vi "create.volume.filename.vi"(11 "volume":T1={"id"=0, "name"="", "sortable_name"="", "aliases"=[], "description"="", "site_detail_url"="", "count_of_issues"=0, "start_year"=0, "publisher_id"=0, "issue_ids"=[], "date_last_updated"=timestamp(0 s since 1904-01-01), "volume"=0, "cv_id"="", "volume type"=enum."One Shot"}) -> (3 "json filename":string)   [LabVIEW 2024]
uses:
  definitions/local_volume.ctl
  definitions/volume.type--enum.ctl
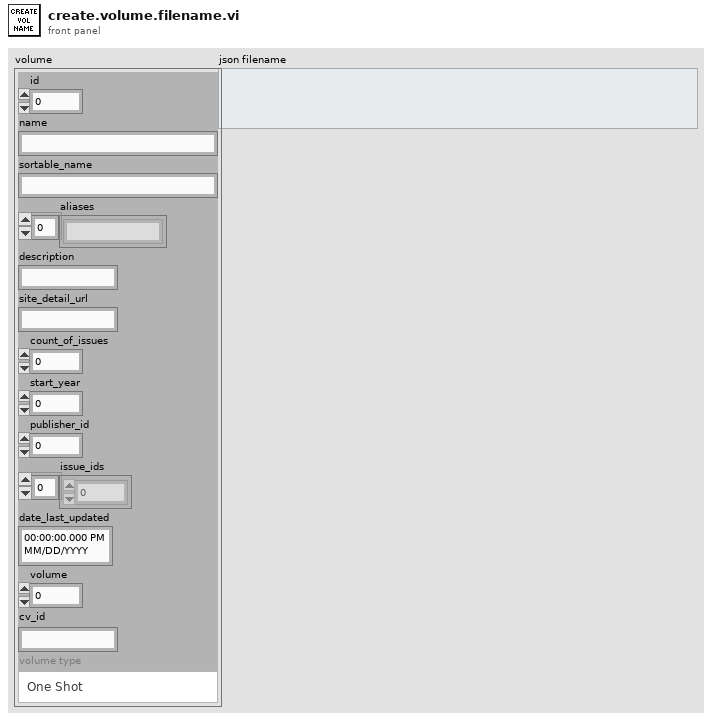
[diagram p1: front panel]
types:
  T1 = typedef "local_volume.ctl" = cluster{"id":i32, "name":string, "sortable_name":string, "aliases":string[], "description":string, "site_detail_url":string, "count_of_issues":i32, "start_year":i32, "publisher_id":i32, "issue_ids":i32[], "date_last_updated":timestamp, "volume":i32, "cv_id":string, "volume type":T2}
  T2 = typedef "volume.type--enum.ctl" = enum16{"Ongoing", "Limited Series", "Annual", "One Shot", "Reprint/Document"}
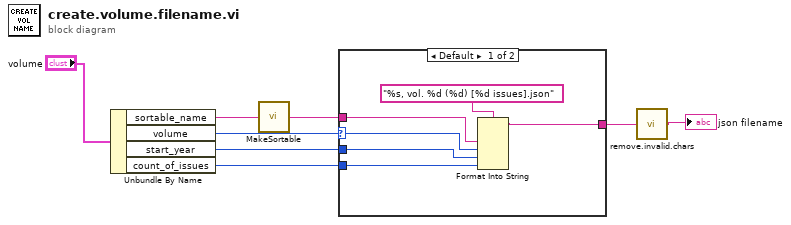
[diagram p0: block diagram]
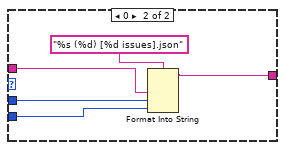
[diagram p2: hidden frame]
diagram:
  n1 = Unbundle By Name("volume") -> ("sortable_name"=w8:string, "volume"=w4:i32, "start_year"=w6:i32, "count_of_issues"=w5:i32)
  n2 = call "MakeSortable.vi"("string in"=w8) -> ("string out"=w7:string)
  n3 = case shown="Default" w4 {
    selector: w4 -> [w9 _]
    tunnel: [w14 w19] -> w3
    tunnel: w7 -> [w12 w17]
    tunnel: w6 -> [w11 w16]
    tunnel: w5 -> [w10 w15]
    frame Default {
      n4 = Format Into String(format string="%s, vol. %d (%d) [%d issues].json", w12, w9, w11, w10) -> (resulting string=w14:string)  [unwired: 2 in, 1 out]
    }
    frame 0 {
      n5 = Format Into String(format string="%s (%d) [%d issues].json", w17, w16, w15) -> (resulting string=w19:string)  [unwired: 2 in, 1 out]
    }
  }
  n6 = call "remove.invalid.chars.vi"("string in"=w3) -> ("string out"=→"json filename":string)
